vi "Handle Response.vi"(8 "error in (no error)":errorcluster, 9 "Abstract Response Message":refnum<class "Abstract Message.lvclass">, 11 "Abstract Producer in":refnum<class "Abstract Producer.lvclass">) -> (0 "error out":errorcluster, 3 "Abstract Producer out":refnum<class "Abstract Producer.lvclass">)   [LabVIEW 2017, in "Messaging.lvlib" / "Abstract Producer.lvclass"]
uses:
  Abstract Producer.lvclass
  Message/Abstract Message/Abstract Message.lvclass
  Message/Abstract Response Message/Abstract Response Message.lvclass
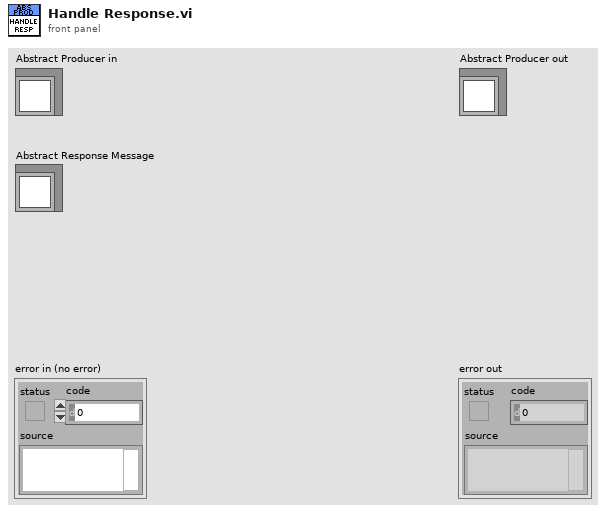
[diagram p1: front panel]
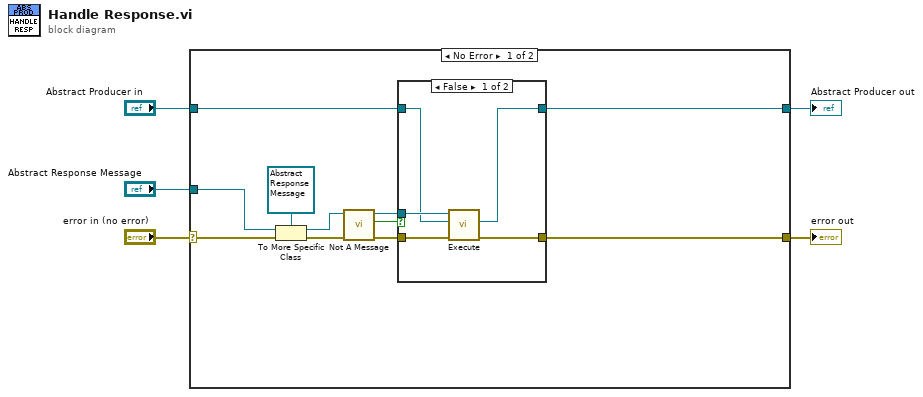
[diagram p0: block diagram]
diagram:
  n1 = case shown="No Error" "error in (no error)" {
    selector: "error in (no error)" -> [w14 w25]
    tunnel: [w6 w25] -> w4
    tunnel: [w7 w24] -> w2
    tunnel: "Abstract Producer in" -> [w8 w24]
    tunnel: "Abstract Response Message" -> [w16 _]
    frame No Error {
      n2 = To More Specific Class(target class=refnum<class "Abstract Response Message.lvclass"> refnum ("Abstract Response Message in"), reference=w16, error in=w14) -> (specific class reference=w12:refnum<class "Abstract Response Message.lvclass">, error out=w13:errorcluster)
      n3 = call "Not A Message.vi"("error in (no error)"=w13, "Abstract Response Message in"=w12) -> ("error out"=w11:errorcluster, "Not a Message?"=w10:bool, "Abstract Response Message out"=w9:refnum<class "Abstract Response Message.lvclass">)  [unwired: 7 in]
      n4 = case shown="False" w10 {
        tunnel: w11 -> [w21 w22]
        tunnel: w9 -> [w20 _]
        tunnel: w8 -> [w19 w23]
        tunnel: [w18 w23] -> w7
        tunnel: [w17 w22] -> w6
        frame False {
          n5 = call-dynamic "Execute.vi"("error in (no error)"=w21, "Abstract Producer in"=w19, "Abstract Response Message in"=w20) -> ("error out"=w17:errorcluster, "Abstract Producer out"=w18:refnum<class "Abstract Producer.lvclass">)  [unwired: 6 in, 1 out]
        }
        frame True {
          # "Nothing to handle"
        }
      }
    }
    frame Error {
    }
  }
  "error out" <- w4
  "Abstract Producer out" <- w2
